vi "Set Sim Parameters GUI.vi"(9 "Scaling":dbl[](array[numeric]), 10 "Offsets":dbl[](array[numeric]), 11 "Channel":string[](array[string])) -> (1 "Scaling out":dbl[](array[numeric]), 2 "Offsets out":dbl[](array[numeric]))   [LabVIEW 2022 SP3, in "Temp Control.lvclass"]
uses:
  Temp Control.lvclass
  Temp Control.lvclass/Temp Control.ctl
panel:
  in  "OK Button":bool
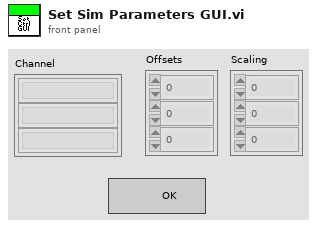
[diagram p1: front panel]
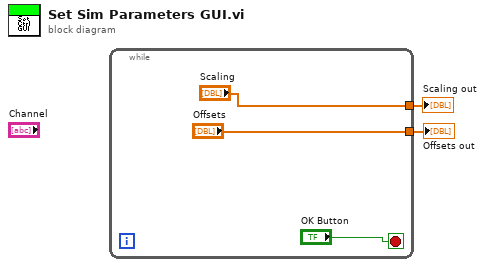
[diagram p0: block diagram]
diagram:
  n1 = while {
    tunnel: ["Scaling"] -> w2
    tunnel: ["Offsets"] -> w1
    stop <- "OK Button" stop-if-true
  }
  "Scaling out" <- w2
  "Offsets out" <- w1
